vi "RDV-testGUI.vi"() -> ()   [LabVIEW 2020, in "RDV-Reflection_Data_viewer.lvclass"]
uses:
  RDV-Reflection_Data_viewer.lvclass
  RDV-PRELAUNCH_DATA.ctl
  RDV-XY_GRAPH_REFS.ctl
  RDV-GUI_REFS.ctl
panel:
  out "error out":errorcluster
  in  "Toggle Visability":bool
  in  "stop":bool
  out "Permittivity Imag":T1(graph)
  out "Permittivity Real":T1(graph)
  out "Reflection Imag":T1(graph)
  out "Reflection Real":T1(graph)
  in  "Folder Path":path=path "C:/projects/Universitet/Master/data/Real Test - First libreVNA test with calibration file/Converted Data"
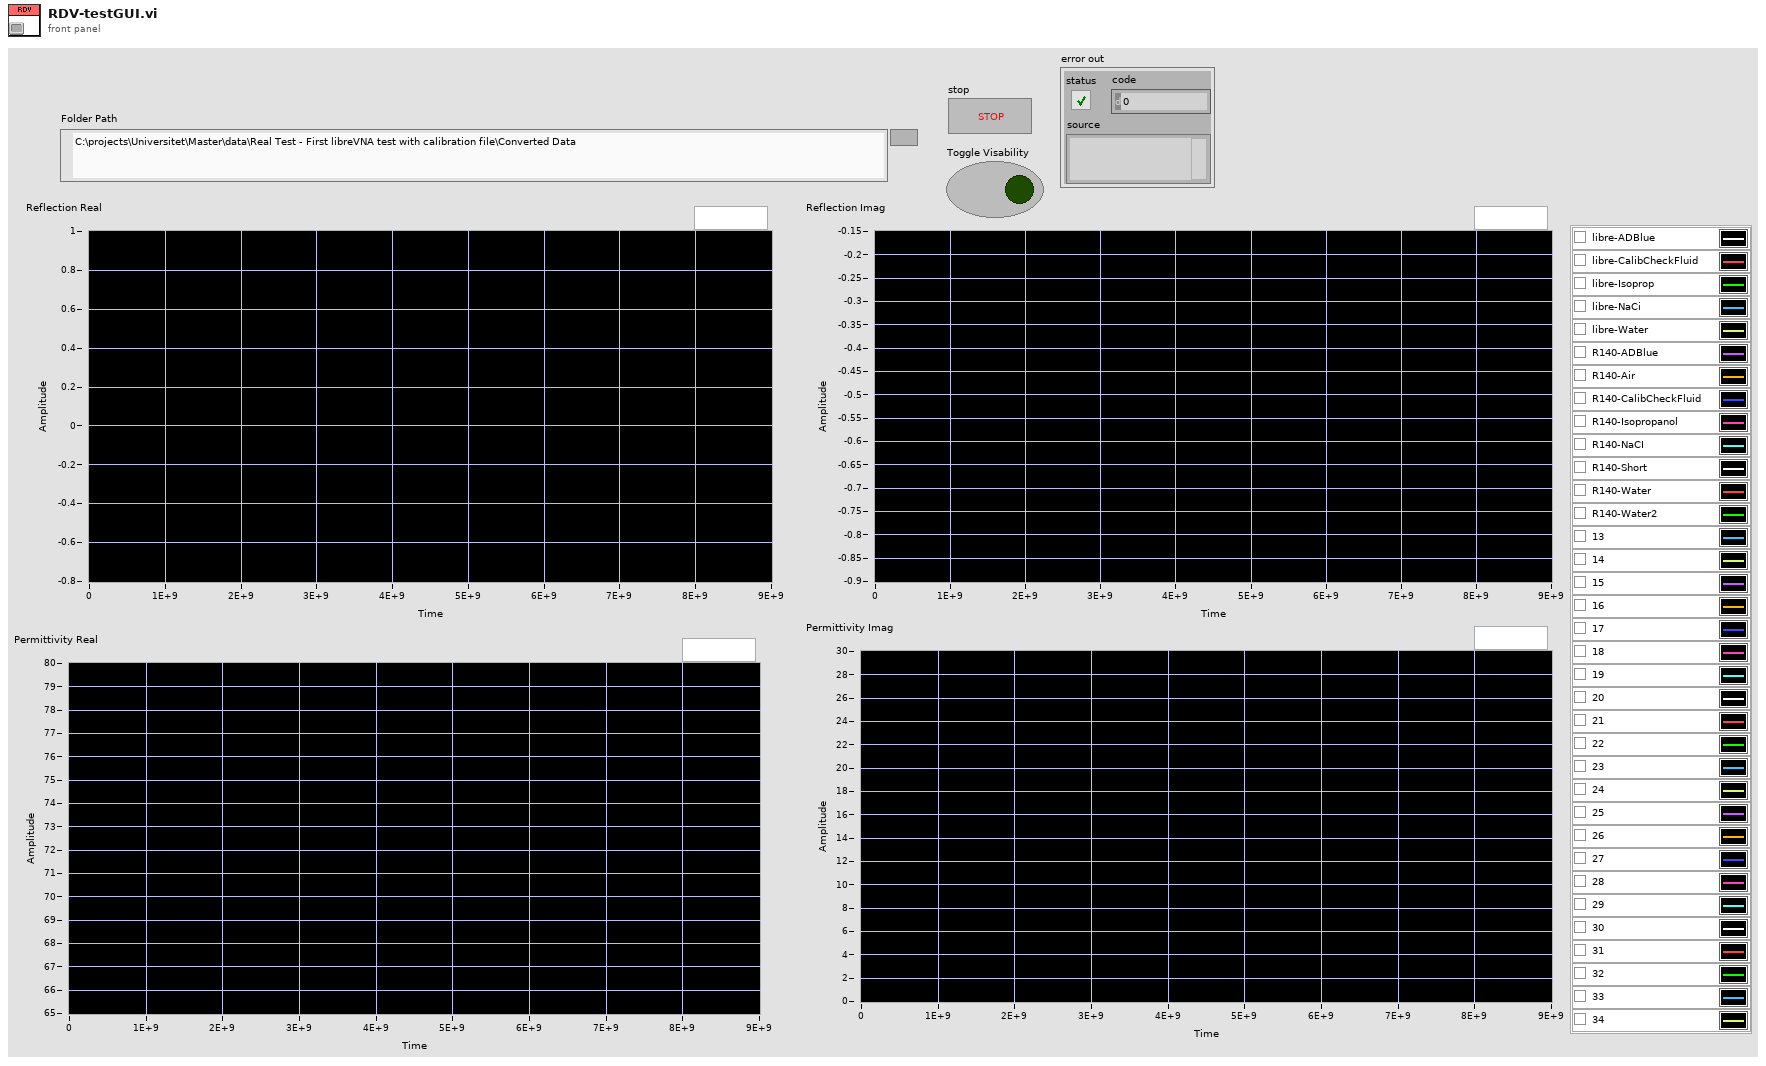
[diagram p1: front panel]
types:
  T1 = cluster{"Frequency":dbl[], "Reflection'":dbl[]}[]
  T2 = typedef "RDV-Reflection_Data_viewer.lvclass/RDV-PRELAUNCH_DATA.ctl" = cluster{"XY graph refs":T3, "GUI Refs":T4}
  T3 = typedef "RDV-Reflection_Data_viewer.lvclass/RDV-XY_GRAPH_REFS.ctl" = cluster{"Reflection Real":refnum<vi>, "Reflection Imag":refnum<vi>, "Permittivity Real":refnum<vi>, "Permittivity Imag":refnum<vi>}
  T4 = typedef "RDV-Reflection_Data_viewer.lvclass/RDV-GUI_REFS.ctl" = cluster{"Autoscale":refnum<vi>, "plot Selector":refnum<vi>[]}
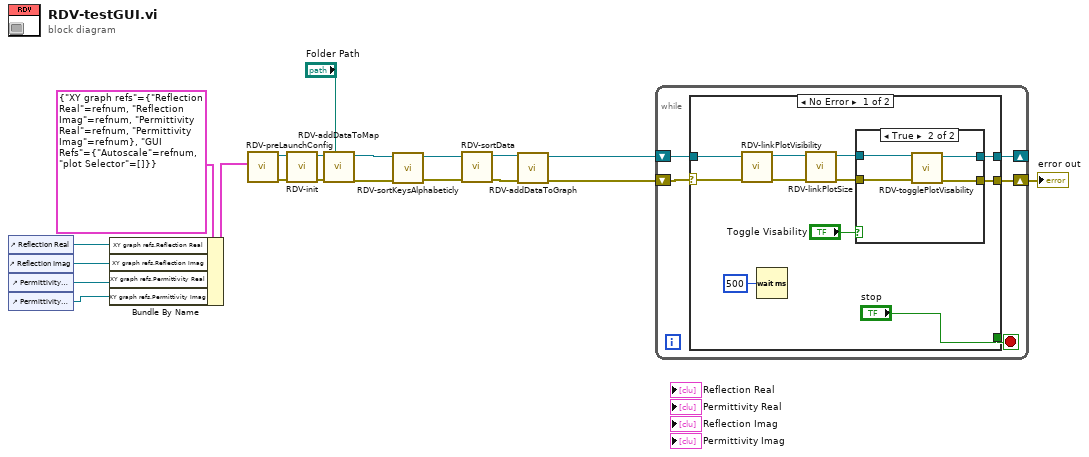
[diagram p0: block diagram]
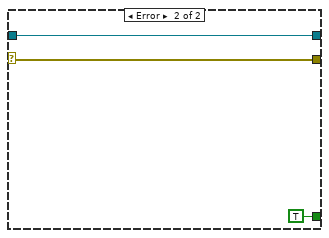
[diagram p3: hidden frame]
diagram:
  n1 = control-ref of="Reflection Real"() -> (w16:refnum<vi>)
  n2 = control-ref of="Reflection Imag"() -> (w15:refnum<vi>)
  n3 = control-ref of="Permittivity Real"() -> (w14:refnum<vi>)
  n4 = control-ref of="Permittivity Imag"() -> (w13:refnum<vi>)
  n5 = Bundle By Name(cluster=T2 {"XY graph refs"={"Reflection Real"=refnum, "Reflection Imag"=refnum, "Permittivity Real"=refnum, "Permittivity Imag"=refnum}, "GUI Refs"={"Autoscale"=refnum, "plot Selector"=[]}} ("preLaunch Config"), "XY graph refs.Reflection Real"=w16, "XY graph refs.Reflection Imag"=w15, "XY graph refs.Permittivity Real"=w14, "XY graph refs.Permittivity Imag"=w13) -> (w5:T2)
  n6 = call "RDV-preLaunchConfig.vi"("preLaunch Config"=w5) -> ("error out"=w1:errorcluster, "RDV-Reflection_Data_viewer out"=w2:refnum<class "RDV-Reflection_Data_viewer.lvclass">)  [unwired: 9 in]
  n7 = call "RDV-init.vi"("error in (no error)"=w1, "RDV-Reflection_Data_viewer in"=w2) -> ("error out"=w3:errorcluster, "RDV-Reflection_Data_viewer out"=w4:refnum<class "RDV-Reflection_Data_viewer.lvclass">)  [unwired: 8 in]
  n8 = call "RDV-addDataToMap.vi"("Folder Path"="Folder Path", "error in (no error)"=w3, "RDV-Reflection_Data_viewer in"=w4) -> ("error out"=w7:errorcluster, "RDV-Reflection_Data_viewer out"=w19:refnum<class "RDV-Reflection_Data_viewer.lvclass">)  [unwired: 7 in]
  n9 = call "RDV-sortKeysAlphabeticly.vi"("error in (no error)"=w7, "RDV-Reflection_Data_viewer in"=w19) -> ("error out"=w8:errorcluster, "RDV-Reflection_Data_viewer out"=w18:refnum<class "RDV-Reflection_Data_viewer.lvclass">)  [unwired: 8 in]
  n10 = call "RDV-sortData.vi"("error in (no error)"=w8, "RDV-Reflection_Data_viewer in"=w18) -> ("error out"=w9:errorcluster, "RDV-Reflection_Data_viewer out"=w12:refnum<class "RDV-Reflection_Data_viewer.lvclass">)  [unwired: 8 in]
  n11 = call "RDV-addDataToGraph.vi"("error in (no error)"=w9, "RDV-Reflection_Data_viewer in"=w12) -> ("error out"=w10:errorcluster, "RDV-Reflection_Data_viewer out"=w11:refnum<class "RDV-Reflection_Data_viewer.lvclass">)  [unwired: 8 in]
  n12 = while {
    shift-right: [w23] -> _
    shift-left: w11 -> [w24]
    shift-right: [w21] -> w6
    shift-left: w10 -> [w22]
    stop <- w25 stop-if-true
    n13 = case shown="No Error" w22 {
      selector: w22 -> [w30 w44]
      tunnel: ["stop" TRUE ("stop")] -> w25
      tunnel: w24 -> [w34 w45]
      tunnel: [w32 w45] -> w23
      tunnel: [w31 w44] -> w21
      frame No Error {
        n14 = call "RDV-linkPlotVisibility.vi"("error in (no error)"=w30, "RDV-Reflection_Data_viewer in"=w34) -> ("error out"=w26:errorcluster, "RDV-Reflection_Data_viewer out"=w29:refnum<class "RDV-Reflection_Data_viewer.lvclass">)  [unwired: 8 in]
        n15 = Wait (ms)(milliseconds to wait=u32 500) -> ()  [unwired: 1 out]
        n16 = call "RDV-linkPlotSize.vi"("error in (no error)"=w26, "RDV-Reflection_Data_viewer in"=w29) -> ("error out"=w27:errorcluster, "RDV-Reflection_Data_viewer out"=w28:refnum<class "RDV-Reflection_Data_viewer.lvclass">)  [unwired: 8 in]
        n17 = case shown="True" "Toggle Visability" {
          tunnel: w28 -> [w38 w42]
          tunnel: [w38 w41] -> w32
          tunnel: [w37 w40] -> w31
          tunnel: w27 -> [w37 w39]
          frame False {
          }
          frame True {
            n18 = call "RDV-togglePlotVisability.vi"("error in (no error)"=w39, "RDV-Reflection_Data_viewer in"=w42) -> ("error out"=w40:errorcluster, "RDV-Reflection_Data_viewer out"=w41:refnum<class "RDV-Reflection_Data_viewer.lvclass">)  [unwired: 8 in]
          }
        }
      }
      frame Error {
      }
    }
  }
  "error out" <- w6
